vi "Ramp Motor Output Test.vi"() -> ()   [LabVIEW 2013]
panel:
  out "Output":dbl(slide) scale=-1.0..1.0
  in  "Input":dbl(slide) scale=-1.0..1.0
  in  "Ramp Time":dbl=250.0 format="%#_13g"
  in  "stop":bool
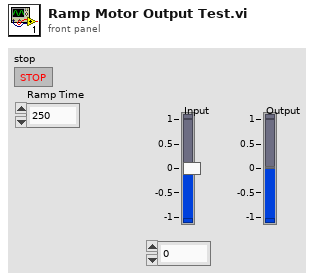
[diagram p1: front panel]
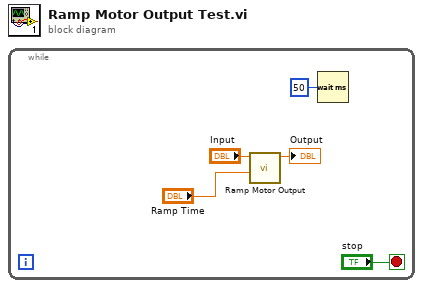
[diagram p0: block diagram]
diagram:
  n1 = while {
    stop <- "stop" stop-if-true
    n2 = call "Ramp Motor Output.vi"("Ramp Time"="Ramp Time", "Input"="Input") -> ("Output"=→"Output":dbl)  [unwired: 9 in]
    n3 = Wait (ms)(milliseconds to wait=u32 50) -> ()  [unwired: 1 out]
  }
